vi "EREG_DIFF.vi"(1 "Target Pressure (psi)":dbl, 2 "data":dynamicdata(waveform)) -> (0 "Output":dbl)   [LabVIEW 2017]
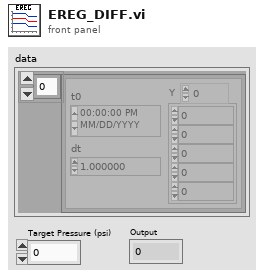
[diagram p1: front panel]
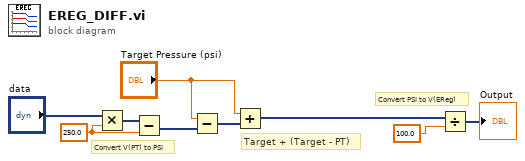
[diagram p0: block diagram]
diagram:
  w6 = 250.0 ("Multiplication factor")
  # "Target + (Target - PT)"
  # "Convert PSI to V(EReg)"
  # "Convert V(PT) to PSI"
  n1 = Multiply(x="data", y=w6) -> (x*y=w7:dynamicdata)
  n2 = Subtract(x=w7, y=w6) -> (x-y=w4:dynamicdata)
  n3 = Subtract(x="Target Pressure (psi)", y=w4) -> (x-y=w3:dynamicdata)
  n4 = Add(x="Target Pressure (psi)", y=w3) -> (x+y=w1:dynamicdata)
  n5 = Divide(x=w1, y=100.0) -> (x/y=→"Output":dynamicdata)
